vi "niDDC Configure Clock.vi"(8 "error in (no error)":errorcluster, 9 "External Clock Frequency (Hz)":dbl=432000000.0 format="%#_6p", 10 "Clock Source":T1(ring)=enum."Internal Clock PLL On (IoModSyncClk)", 11 "Class in":refnum<class "7976R_v1.lvclass">) -> (0 "error out":errorcluster, 3 "Class out":refnum<class "7976R_v1.lvclass">)   [LabVIEW 2015, in "7976R_v1.lvclass"]
uses:
  <userlib>/SE-APP-Receiver/NI5772/7976R_v1/7976R_v1.lvclass
  <userlib>/SE-APP-Receiver/NI5772/7976R_v1/7976R_v1.lvclass/7976R_v1.ctl
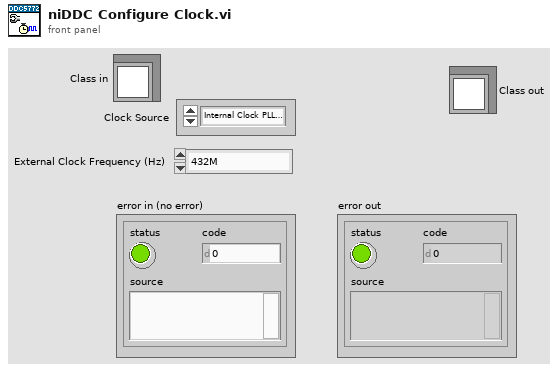
[diagram p1: front panel]
types:
  T1 = enum8{"Internal Clock PLL Off", "Internal Clock PLL On (REF IN)", "External Clock (CLK_IN)", "Internal Clock PLL On (IoModSyncClk)"}
  T2 = typedef "7976R_v1.lvclass/FPGA VI Reference_DDC_v1.8.ctl" = refnum<k20>
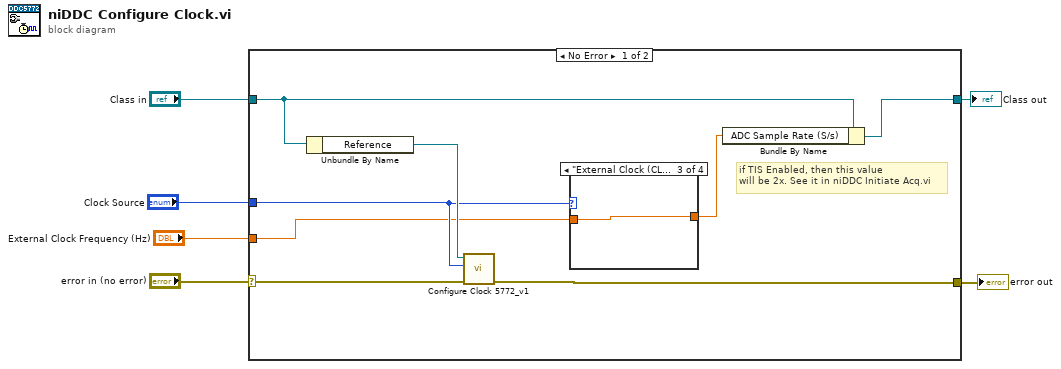
[diagram p0: block diagram]
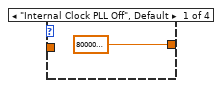
[diagram p2: hidden frame]
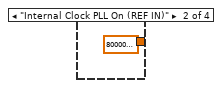
[diagram p3: hidden frame]
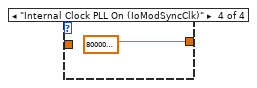
[diagram p4: hidden frame]
diagram:
  n1 = case shown="No Error" "error in (no error)" {
    selector: "error in (no error)" -> [w13 w19]
    tunnel: [w12 w19] -> w6
    tunnel: "Class in" -> [w9 w20]
    tunnel: [w8 w20] -> w3
    tunnel: "Clock Source" -> [w11 _]
    tunnel: "External Clock Frequency (Hz)" -> [w10 _]
    frame No Error {
      # "if TIS Enabled, then this value\nwill be 2x. See it in niDDC Initiate Acq.vi"
      n2 = Unbundle By Name(w9) -> ("Reference"=w14:T2)
      n3 = call <userlib>:"Configure Clock 5772_v1.vi"("error in"=w13, "Clock Source"=w11, "FPGA VI Reference In"=w14) -> ("error out"=w12:errorcluster)  [unwired: 6 in, 2 out]
      n4 = case shown="\"External Clock (CLK_IN)\"" w11 {
        tunnel: w10 -> [_ _ w17 _]
        tunnel: [800000000.0 ("External Clock Frequency (Hz)") 800000000.0 ("External Clock Frequency (Hz)") w17 800000000.0 ("External Clock Frequency (Hz)")] -> w7
        frame "Internal Clock PLL Off", Default {
        }
        frame "Internal Clock PLL On (REF IN)" {
        }
        frame "External Clock (CLK_IN)" {
        }
        frame "Internal Clock PLL On (IoModSyncClk)" {
        }
      }
      n5 = Bundle By Name(cluster=w9, "ADC Sample Rate (S/s)"=w7) -> (w8:refnum<class "7976R_v1.lvclass">)
    }
    frame Error {
    }
  }
  "error out" <- w6
  "Class out" <- w3
